vi "Write Channel.vi"(8 "error in (no error)":errorcluster, 10 "Channel":refnum<vi>, 11 "Analog-Output in":refnum<class "Analog-Output.lvclass">) -> (0 "error out":errorcluster, 3 "Analog-Output out":refnum<class "Analog-Output.lvclass">)   [LabVIEW 2019, in "Analog-Output.lvlib" / "Analog-Output.lvclass"]
uses:
  Library/Analog-Output.lvclass
  Library/Analog-Output.lvclass/Analog-Output.ctl
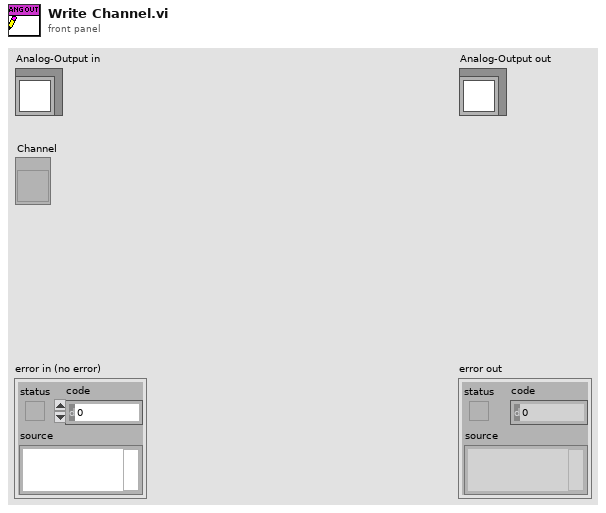
[diagram p1: front panel]
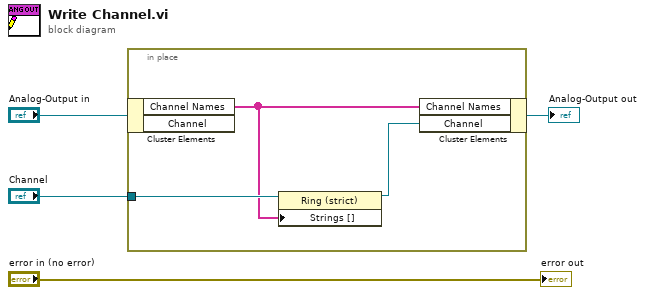
[diagram p0: block diagram]
diagram:
  n1 = in-place {
    in-place-border: "Channel" -> [w7]
    n2 = in-place-cluster #1("Analog-Output in") -> ("Channel Names"=w6:string[])  [unwired: 1 out]
    n3 = property class="Ring (strict)"(reference=w7, "Strings []"=w6) -> (reference out=w5:refnum<vi>)  [unwired: 1 in, 1 out]
    n4 = in-place-cluster #1("Channel Names"=w6, "Channel"=w5) -> (→"Analog-Output out":refnum<class "Analog-Output.lvclass">)
  }
  "error out" <- "error in (no error)"
